vi "Convert Network Parameters.vi"(7 "Parameters to convert":enum16{"Y", "Z", "T"}(ring), 8 "error in (no error)":errorcluster, 10 "Zc (Ohm)":cdb[](array[numeric]), 11 "S-par Array In":cdb[][](array[numeric])) -> (0 "error out":errorcluster, 2 "Yc/Zc":cdb[](array[numeric]), 3 "Y/Z Array Out":cdb[][](array[numeric]))   [LabVIEW 2020]
uses:
  <vilib>/addons/HF Network Analysis/NI_HFNetworkAnalysis.lvlib
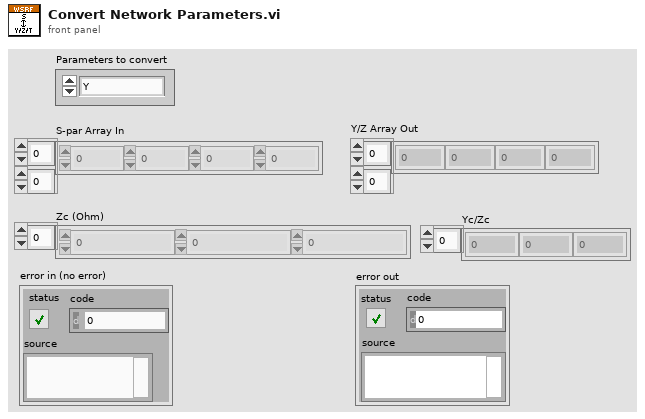
[diagram p1: front panel]
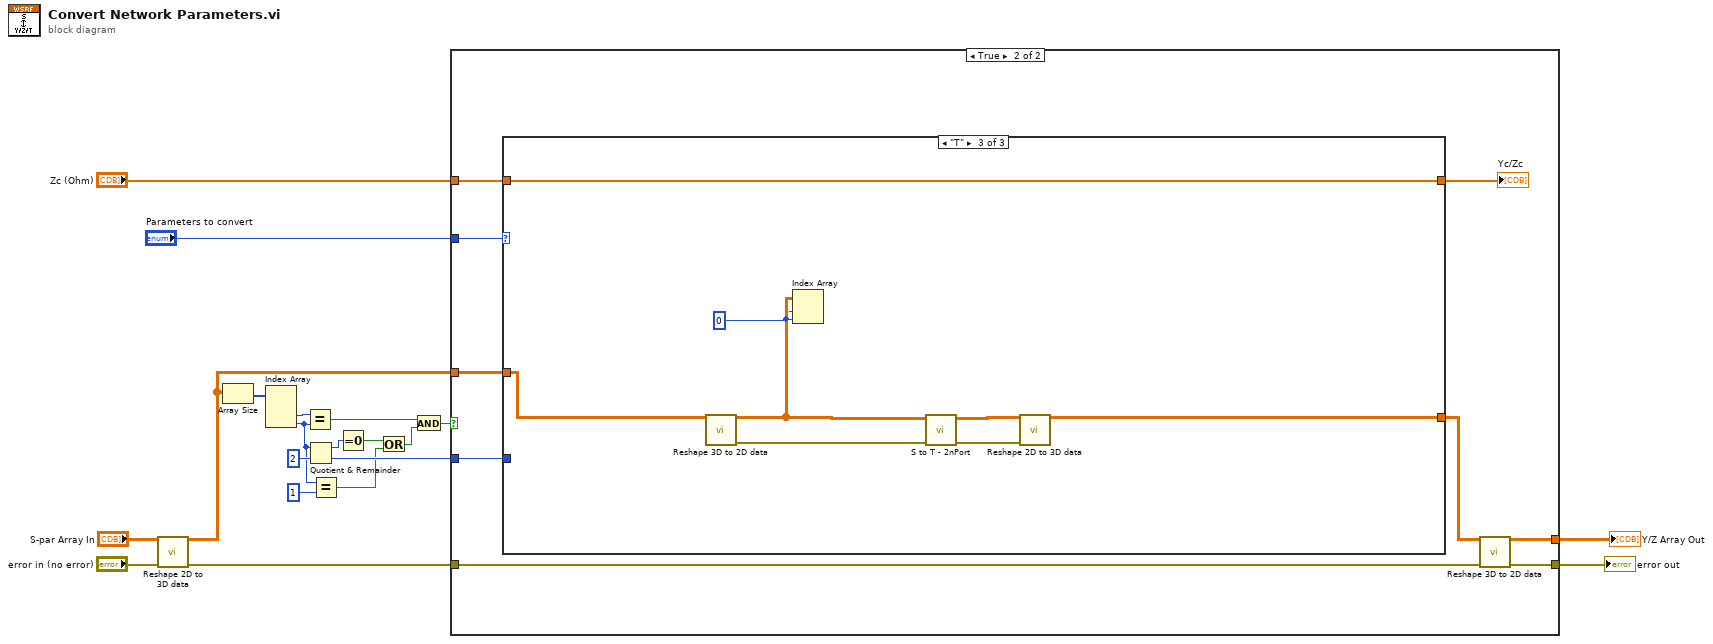
[diagram p0: block diagram]
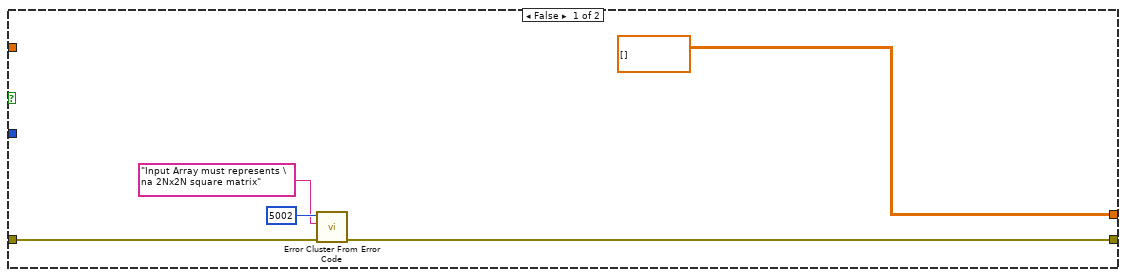
[diagram p2: hidden frame]
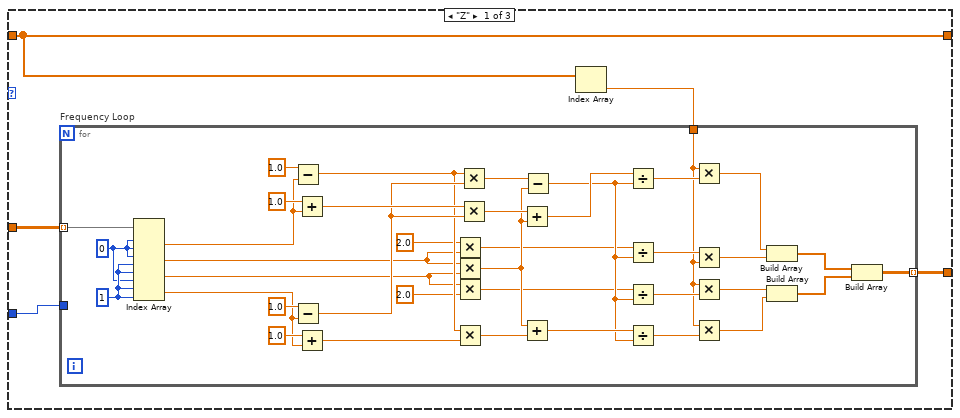
[diagram p3: hidden frame]
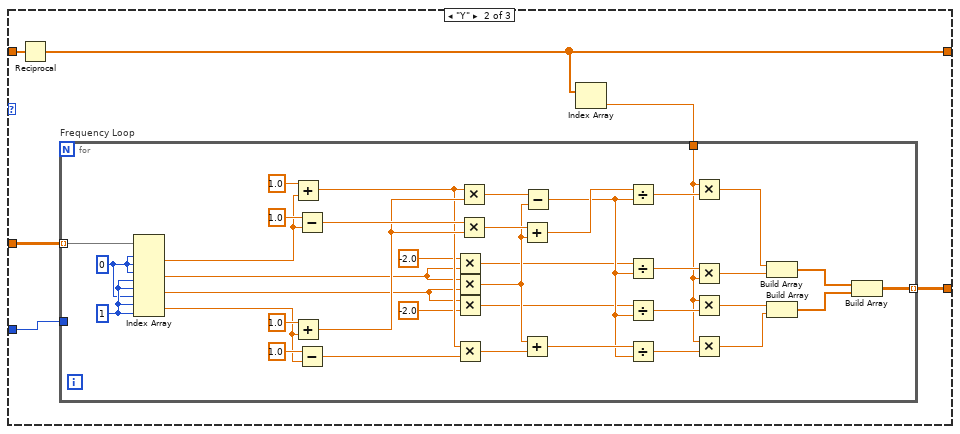
[diagram p4: hidden frame]
diagram:
  n1 = call <vilib>:"Reshape 2D to 3D data.vi"("Parameters In (2D)"="S-par Array In", "Error In"="error in (no error)") -> ("Parameters Out (3D)"=w19:cdb[][][], "Error Out"=w13:errorcluster)  [unwired: 12 in]
  n2 = Array Size(array=w19) -> (size(s)=w18:i32[])
  n3 = Index Array(array=w18) -> (element #2=w8:i32, element #3=w2:i32)  [unwired: 3 in, 1 out]
  n4 = Equal?(x=w8, y=w2) -> (x = y?=w16:bool)
  n5 = Quotient & Remainder(x=w2, y=2) -> (x-y*floor(x/y)=w10:i32, floor(x/y)=w9:i32)
  n6 = Equal?(x=w2, y=1) -> (x = y?=w3:bool)
  n7 = Equal To 0?(x=w10) -> (x = 0?=w5:bool)
  n8 = Or(x=w5, y=w3) -> (x .or. y?=w4:bool)
  n9 = And(x=w16, y=w4) -> (x .and. y?=w15:bool)
  n10 = case shown="True" w15 {
    tunnel: w19 -> [_ w34]
    tunnel: w9 -> [_ w33]
    tunnel: [cdb[][] [] ("Parameters Out (2D)") w32] -> w14
    tunnel: w13 -> [w24 w30]
    tunnel: [w23 w31] -> w11
    tunnel: "Zc (Ohm)" -> [_ w27]
    tunnel: "Parameters to convert" -> [_ w26]
    frame False {
      n11 = call <vilib>:"Error Cluster From Error Code.vi"("error in (no error)"=w24, "error message (\"\")"="Input Array must represents \na 2Nx2N square matrix" ("error message (\"\")"), "error code (0)"=5002) -> ("error out"=w23:errorcluster)  [unwired: 6 in]
    }
    frame True {
      n12 = case shown="\"T\"" w26 {
        tunnel: w34 -> [w39 w83 w129]
        tunnel: w33 -> [w38 w82 _]
        tunnel: [w37 w81 w126] -> w29
        tunnel: [w36 w80 w124] -> w28
        tunnel: w27 -> [w36 w79 w124]
        frame "Z" {
          n13 = Index Array(array=w36) -> (element=w35:cdb)  [unwired: 1 in]
          n14 = for "Frequency Loop" {
            tunnel: w39 -> [w41] mode=indexing
            tunnel: w38 -> [_]
            tunnel: [w40] -> w37 mode=indexing
            tunnel: w35 -> [w48]
            w77 = 1 ("index (row)")
            w76 = 0 ("index (row)")
            n15 = Index Array(array=w41, index (row) #1=w76, index (col) #1=w76, index (row) #2=w76, index (col) #2=w77, index (row) #3=w77, index (col) #3=w76, index (row) #4=w77, index (col) #4=w77) -> (element #1=w70:cdb, element #2=w54:cdb, element #3=w56:cdb, element #4=w64:cdb)
            n16 = Subtract(x=1.0, y=w70) -> (x-y=w62:cdb)
            n17 = Subtract(x=1.0, y=w64) -> (x-y=w68:cdb)
            n18 = Add(x=1.0, y=w70) -> (x+y=w73:cdb)
            n19 = Add(x=1.0, y=w64) -> (x+y=w61:cdb)
            n20 = Multiply(x=2.0, y=w54) -> (x*y=w52:cdb)
            n21 = Multiply(x=w54, y=w56) -> (x*y=w63:cdb)
            n22 = Multiply(x=w56, y=2.0) -> (x*y=w51:cdb)
            n23 = Multiply(x=w62, y=w61) -> (x*y=w60:cdb)
            n24 = Multiply(x=w62, y=w68) -> (x*y=w67:cdb)
            n25 = Multiply(x=w73, y=w68) -> (x*y=w72:cdb)
            n26 = Add(x=w72, y=w63) -> (x+y=w69:cdb)
            n27 = Add(x=w63, y=w60) -> (x+y=w59:cdb)
            n28 = Subtract(x=w67, y=w63) -> (x-y=w53:cdb)
            n29 = Divide(x=w69, y=w53) -> (x/y=w66:cdb)
            n30 = Divide(x=w52, y=w53) -> (x/y=w49:cdb)
            n31 = Divide(x=w51, y=w53) -> (x/y=w50:cdb)
            n32 = Divide(x=w59, y=w53) -> (x/y=w58:cdb)
            n33 = Multiply(x=w48, y=w66) -> (x*y=w47:cdb)
            n34 = Multiply(x=w49, y=w48) -> (x*y=w46:cdb)
            n35 = Multiply(x=w48, y=w50) -> (x*y=w44:cdb)
            n36 = Multiply(x=w48, y=w58) -> (x*y=w43:cdb)
            n37 = Build Array(w47, w46) -> (w45:cdb[])
            n38 = Build Array(w44, w43) -> (w42:cdb[])
            n39 = Build Array(w45, w42) -> (w40:cdb[][])
          }
        }
        frame "Y" {
          n40 = Reciprocal(x=w79) -> (1/x=w80:cdb[])
          n41 = Index Array(array=w80) -> (element=w78:cdb)  [unwired: 1 in]
          n42 = for "Frequency Loop" {
            tunnel: w83 -> [w85] mode=indexing
            tunnel: w82 -> [_]
            tunnel: [w84] -> w81 mode=indexing
            tunnel: w78 -> [w92]
            w121 = 1 ("index (row)")
            w120 = 0 ("index (row)")
            n43 = Index Array(array=w85, index (row) #1=w120, index (col) #1=w120, index (row) #2=w120, index (col) #2=w121, index (row) #3=w121, index (col) #3=w120, index (row) #4=w121, index (col) #4=w121) -> (element #1=w114:cdb, element #2=w98:cdb, element #3=w100:cdb, element #4=w108:cdb)
            n44 = Add(x=1.0, y=w114) -> (x+y=w106:cdb)
            n45 = Add(x=1.0, y=w108) -> (x+y=w112:cdb)
            n46 = Subtract(x=1.0, y=w114) -> (x-y=w117:cdb)
            n47 = Subtract(x=1.0, y=w108) -> (x-y=w105:cdb)
            n48 = Multiply(x=-2.0, y=w98) -> (x*y=w96:cdb)
            n49 = Multiply(x=w98, y=w100) -> (x*y=w107:cdb)
            n50 = Multiply(x=w100, y=-2.0) -> (x*y=w95:cdb)
            n51 = Multiply(x=w106, y=w105) -> (x*y=w104:cdb)
            n52 = Multiply(x=w106, y=w112) -> (x*y=w111:cdb)
            n53 = Multiply(x=w117, y=w112) -> (x*y=w116:cdb)
            n54 = Add(x=w116, y=w107) -> (x+y=w113:cdb)
            n55 = Add(x=w107, y=w104) -> (x+y=w103:cdb)
            n56 = Subtract(x=w111, y=w107) -> (x-y=w97:cdb)
            n57 = Divide(x=w113, y=w97) -> (x/y=w110:cdb)
            n58 = Divide(x=w96, y=w97) -> (x/y=w93:cdb)
            n59 = Divide(x=w95, y=w97) -> (x/y=w94:cdb)
            n60 = Divide(x=w103, y=w97) -> (x/y=w102:cdb)
            n61 = Multiply(x=w92, y=w110) -> (x*y=w91:cdb)
            n62 = Multiply(x=w93, y=w92) -> (x*y=w90:cdb)
            n63 = Multiply(x=w92, y=w94) -> (x*y=w88:cdb)
            n64 = Multiply(x=w92, y=w102) -> (x*y=w87:cdb)
            n65 = Build Array(w91, w90) -> (w89:cdb[])
            n66 = Build Array(w88, w87) -> (w86:cdb[])
            n67 = Build Array(w89, w86) -> (w84:cdb[][])
          }
        }
        frame "T" {
          w122 = 0 ("disabled index (col)")
          n68 = call <vilib>:"Reshape 3D to 2D data.vi"("Parameters In (3D)"=w129) -> ("Parameters Out (2D)"=w123:cdb[][], "Error Out"=w128:errorcluster)  [unwired: 13 in]
          n69 = Index Array(array=w123, index (row)=w122, index (col)=w122) -> ()  [unwired: 1 out]
          n70 = call <vilib>:"S to T - 2nPort.vi"("error in (no error)"=w128, "S-par Array In"=w123) -> ("error out"=w125:errorcluster, "T-par Array Out"=w127:cdb[][])  [unwired: 8 in]
          n71 = call <vilib>:"Reshape 2D to 3D data.vi"("Parameters In (2D)"=w127, "Error In"=w125) -> ("Parameters Out (3D)"=w126:cdb[][][])  [unwired: 12 in, 1 out]
        }
      }
      "Yc/Zc" <- w28
      n72 = call <vilib>:"Reshape 3D to 2D data.vi"("Parameters In (3D)"=w29, "Error In"=w30) -> ("Parameters Out (2D)"=w32:cdb[][], "Error Out"=w31:errorcluster)  [unwired: 12 in]
    }
  }
  "Y/Z Array Out" <- w14
  "error out" <- w11
